vi "GetOptimalPacketSize.vi"(4 "error in (no error)":errorcluster, 7 "nInputHandle":u64) -> (0 "error out":errorcluster, 1 "GX_STATUS":i32, 2 "punPacketSize":i32, 3 "nOutputHandle":u64)   [LabVIEW 2016, in "GxLVLib.lvlib"]
uses:
  GxLVLib.lvlib
  GxIAPI.dll
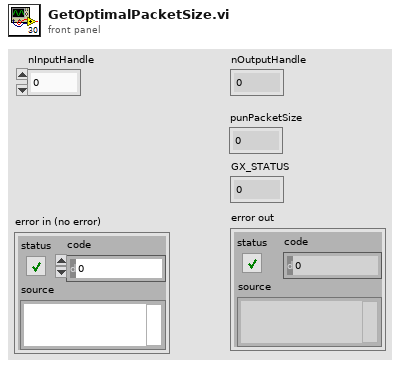
[diagram p1: front panel]
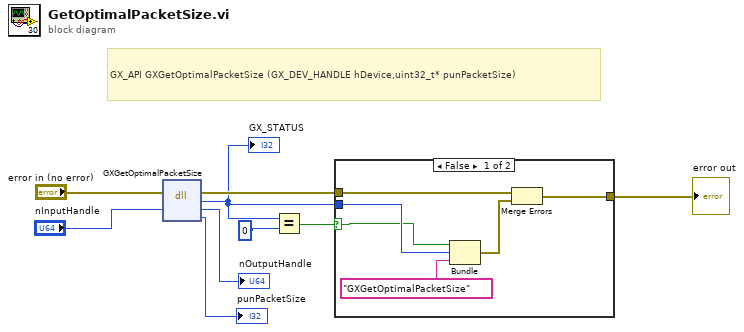
[diagram p0: block diagram]
diagram:
  # "GX_API GXGetOptimalPacketSize (GX_DEV_HANDLE hDevice,uint32_t* punPacketSize)"
  n1 = dll-call lib="GxIAPI.dll" fn="GXGetOptimalPacketSize"(error in="error in (no error)", "hDevice"="nInputHandle") -> (error out=w5:errorcluster, "GX_STATUS"=w2:i32, "hDevice"=→"nOutputHandle":i64, "punPacketSize"=→"punPacketSize":i32)  [unwired: 3 in, 1 out]
  "GX_STATUS" <- w2
  n2 = Equal?(x=w2, y=0) -> (x = y?=w4:bool)
  n3 = case shown="False" w4 {
    selector: w4 -> [w11 _]
    tunnel: w5 -> [w15 w16]
    tunnel: [w14 w16] -> w6
    tunnel: w2 -> [w12 _]
    frame False {
      n4 = Bundle(w11, "GX_STATUS"=w12, "GXGetOptimalPacketSize") -> (w13:cluster{bool, "GX_STATUS":i32, string})  [unwired: 1 in]
      n5 = Merge Errors(w15, w13) -> (w14:errorcluster)
    }
    frame True {
    }
  }
  "error out" <- w6
